vi "Enum Select.vi"(9 "Values":u16[](array[numeric]), 10 "Selections":string[](array[string]), 11 "Select Message":string) -> (1 "Selected":u16, 3 "Cancelled":bool)   [LabVIEW 2019, in "Test Selector.lvlib" / "Test Selector.lvclass"]
uses:
  Test Selector.lvclass
panel:
  in  "Cancel":bool
  in  "Ring":u16(ring)
  in  "OK":bool
  out "String":string
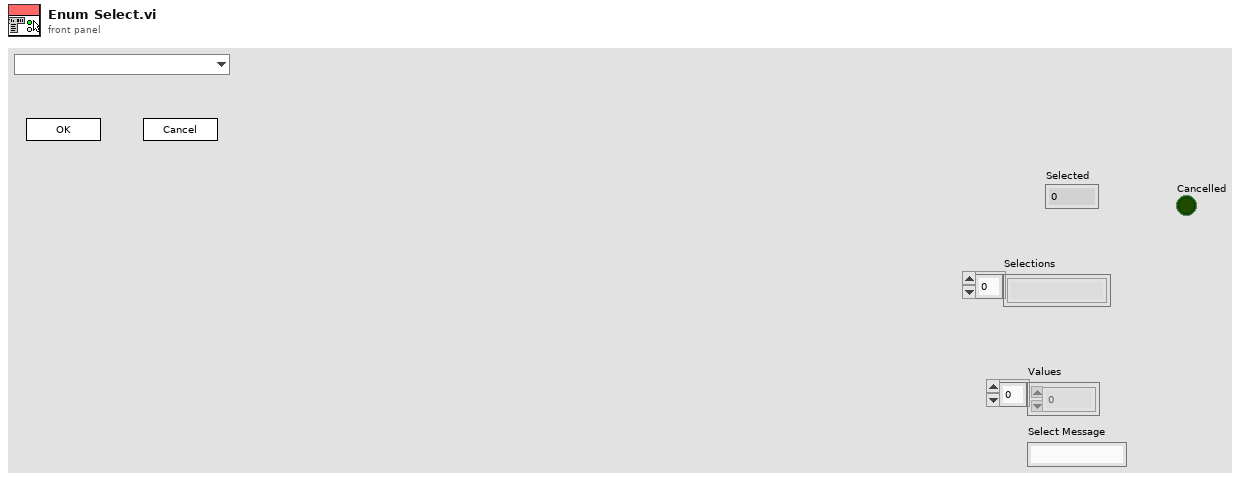
[diagram p1: front panel]
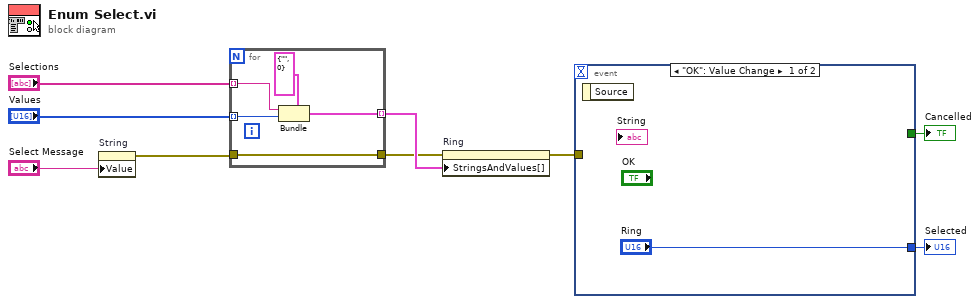
[diagram p0: block diagram]
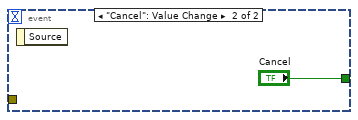
[diagram p2: hidden frame]
diagram:
  n1 = property on="String" class="Str"("Value"="Select Message") -> (error out=w5:errorcluster)  [unwired: 2 in, 1 out]
  n2 = for {
    tunnel: [w12] -> w9 mode=indexing
    tunnel: w5 -> [w11]
    tunnel: "Selections" -> [w13] mode=indexing
    tunnel: "Values" -> [w14] mode=indexing
    tunnel: [w11] -> w1
    n3 = Bundle(cluster=cluster{"String":string, "Value":u16} {"String"="", "Value"=0} ("element"), "String"=w13, "Value"=w14) -> (w12:cluster{"String":string, "Value":u16})
  }
  n4 = property on="Ring" class="Ring (strict)"(error in=w1, "StringsAndValues[]"=w9) -> (error out=w6:errorcluster)  [unwired: 1 in, 1 out]
  n5 = event shown="[0] \"OK\": Value Change" {
    selector: _ -> [_ _]
    dyn-events: _ -> [_ _]
    timeout: _ -> [_ _]
    tunnel: w6 -> [_ _]
    tunnel: ["Ring" _] -> w7
    tunnel: [_ "Cancel"] -> w8
    event "OK": Value Change {
      n6 = event-data() -> ()  [unwired: 1 in, 1 out]
    }
    event "Cancel": Value Change {
      n7 = event-data() -> ()  [unwired: 1 in, 1 out]
    }
  }
  "Selected" <- w7
  "Cancelled" <- w8
